vi "Single Channel Temp Configure Thermocouple.vi"(6 "Channel":string, 7 "SampTime":dbl, 8 "error in (no error)":errorcluster {"code" format="%.0x"}, 9 "SampCount":i32 format="%.0g", 10 "ThermocoupleType (B)":i32(ring) items=["B", "E", "J", "K", "N", "r", "S", "T"], 11 "instrument handle":refnum<k15>) -> (0 "error out":errorcluster {"code" format="%.0x"}, 3 "instrument handle out":refnum<k15>)   [LabVIEW 2020, in "Keysight DAQ970.lvlib"]
doc: "Configures a single channel for thermocouple temperature DMM digitizing, but they do not initiate the digitizing. This command redefines the scan list."
uses:
  Keysight DAQ970.lvlib
  KtDAQ970.dll
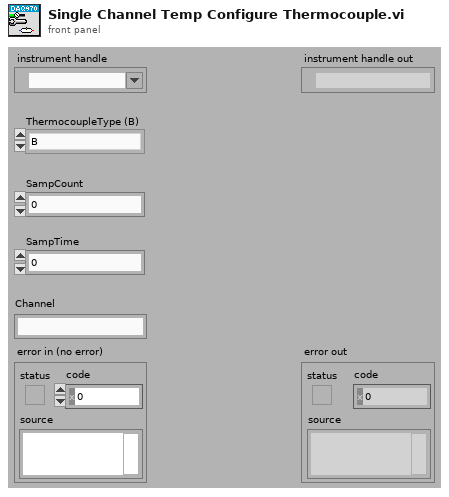
[diagram p1: front panel]
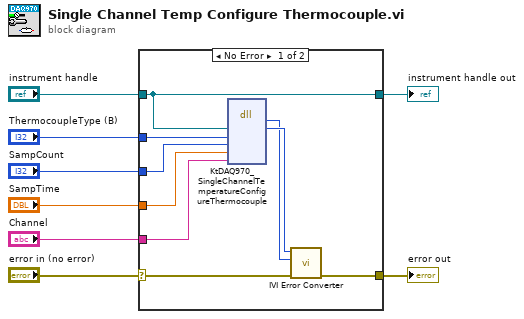
[diagram p0: block diagram]
diagram:
  n1 = case shown="No Error" "error in (no error)" {
    selector: "error in (no error)" -> [w15 w19]
    tunnel: [w14 w19] -> w8
    tunnel: "instrument handle" -> [w9 w18]
    tunnel: "ThermocoupleType (B)" -> [w13 _]
    tunnel: "SampCount" -> [w12 _]
    tunnel: "SampTime" -> [w11 _]
    tunnel: "Channel" -> [w10 _]
    tunnel: [w9 w18] -> w1
    frame No Error {
      n2 = dll-call lib="KtDAQ970**.dll" fn="KtDAQ970_SingleChannelTemperatureConfigureThermocouple"("Vi"=w9, "ThermocoupleType"=w13, "SampCount"=w12, "SampTime"=w11, "Channel"=w10) -> (w16:i32, "Vi"=w17:u32)  [unwired: 7 in, 2 out]
      n3 = call "IVI Error Converter.vi"("error in (no error)"=w15, "IVI error code (0)"=w16, "instrument handle"=w17) -> ("error out"=w14:errorcluster)  [unwired: 7 in, 1 out]
    }
    frame Error {
    }
  }
  "error out" <- w8
  "instrument handle out" <- w1
